vi "OffsetUsingPickRotateDrop.vi"() -> ()   [LabVIEW 2019]
panel:
  in  "DropPlate":i32=2162688
  in  "PickPlate":u32=52428800
  in  "Z":dbl=65.0
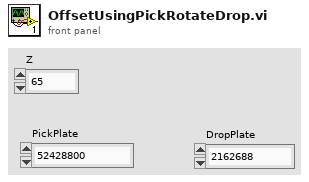
[diagram p1: front panel]
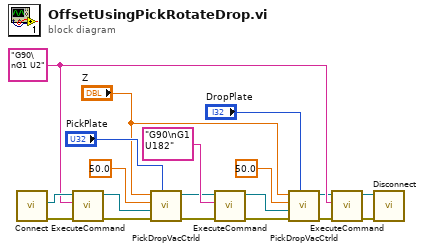
[diagram p0: block diagram]
diagram:
  w5 = "G90\nG1 U2"
  n1 = call "Connect.vi"() -> ("error out"=w17:errorcluster, "controller"=w16:refnum<k24>)  [unwired: 10 in]
  n2 = call "ExecuteCommand.vi"("error in (no error)"=w17, "Command Code"=w5, "controller in"=w16) -> ("error out"=w14:errorcluster, "controller out"=w15:refnum<k24>)  [unwired: 6 in, 1 out]
  n3 = call "PickDropVacCtrld.vi"("VacuumState"="PickPlate", "error in (no error)"=w14, "controller in"=w15, "Zspeed"=50.0, "Z"="Z") -> ("error out"=w12:errorcluster, "controller out"=w11:refnum<k24>)  [unwired: 5 in]
  n4 = call "ExecuteCommand.vi"("error in (no error)"=w12, "Command Code"="G90\nG1 U182", "controller in"=w11) -> ("error out"=w6:errorcluster, "controller out"=w7:refnum<k24>)  [unwired: 6 in, 1 out]
  n5 = call "PickDropVacCtrld.vi"("VacuumState"="DropPlate", "error in (no error)"=w6, "controller in"=w7, "Zspeed"=50.0, "Z"="Z") -> ("error out"=w4:errorcluster, "controller out"=w3:refnum<k24>)  [unwired: 5 in]
  n6 = call "ExecuteCommand.vi"("error in (no error)"=w4, "Command Code"=w5, "controller in"=w3) -> ("error out"=w1:errorcluster, "controller out"=w2:refnum<k24>)  [unwired: 6 in, 1 out]
  n7 = call "Disconnect.vi"("error in (no error)"=w1, "controller"=w2) -> ()  [unwired: 9 in, 1 out]
